vi "Quit.vi"(6 "Operation":T1, 8 "Error In":errorcluster, 9 "Quit":bool) -> (0 "Error Out":errorcluster, 1 "Quit?":bool)   [LabVIEW 2020]
uses:
  Global Variable Operation.ctl
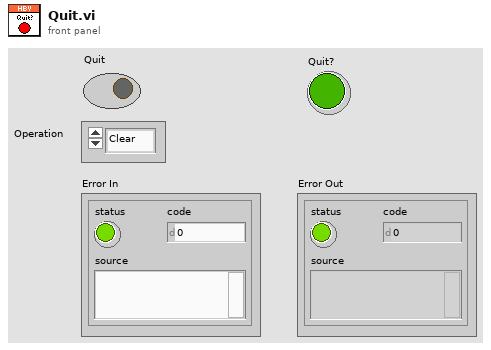
[diagram p1: front panel]
types:
  T1 = typedef "Global Variable Operation.ctl" = enum16{"Clear", "Set", "Get"}
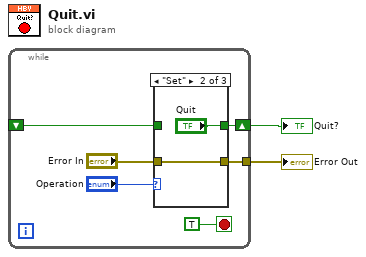
[diagram p0: block diagram]
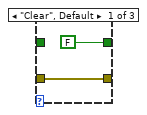
[diagram p2: hidden frame]
diagram:
  n1 = while {
    shift-right: [w7] -> w2
    shift-left: _ -> [w6]
    tunnel: [w3] -> w1
    stop <- TRUE stop-if-true
    n2 = case shown="\"Set\"" "Operation" {
      tunnel: [FALSE ("T button?") "Quit" w14] -> w7
      tunnel: w6 -> [_ _ w14]
      tunnel: "Error In" -> [w9 w11 w13]
      tunnel: [w9 w11 w13] -> w3
      frame "Clear", Default {
      }
      frame "Set" {
      }
      frame "Get" {
      }
    }
  }
  "Error Out" <- w1
  "Quit?" <- w2
